vi "sha256.vi"(11 "data":string) -> (3 "sha256":u32[](array[numeric]) format="%08x")   [LabVIEW 2020, in "wamplv.lvlib" / "HashLib.lvclass"]
doc: "Calculates the <b>SHA-256</b> hash of the <b>data</b> input string.\n\nRFC 4634\n\nCreated by: Ryan Pacini"
uses:
  HashLib.lvclass
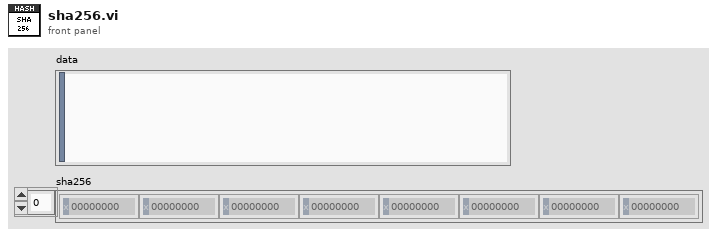
[diagram p1: front panel]
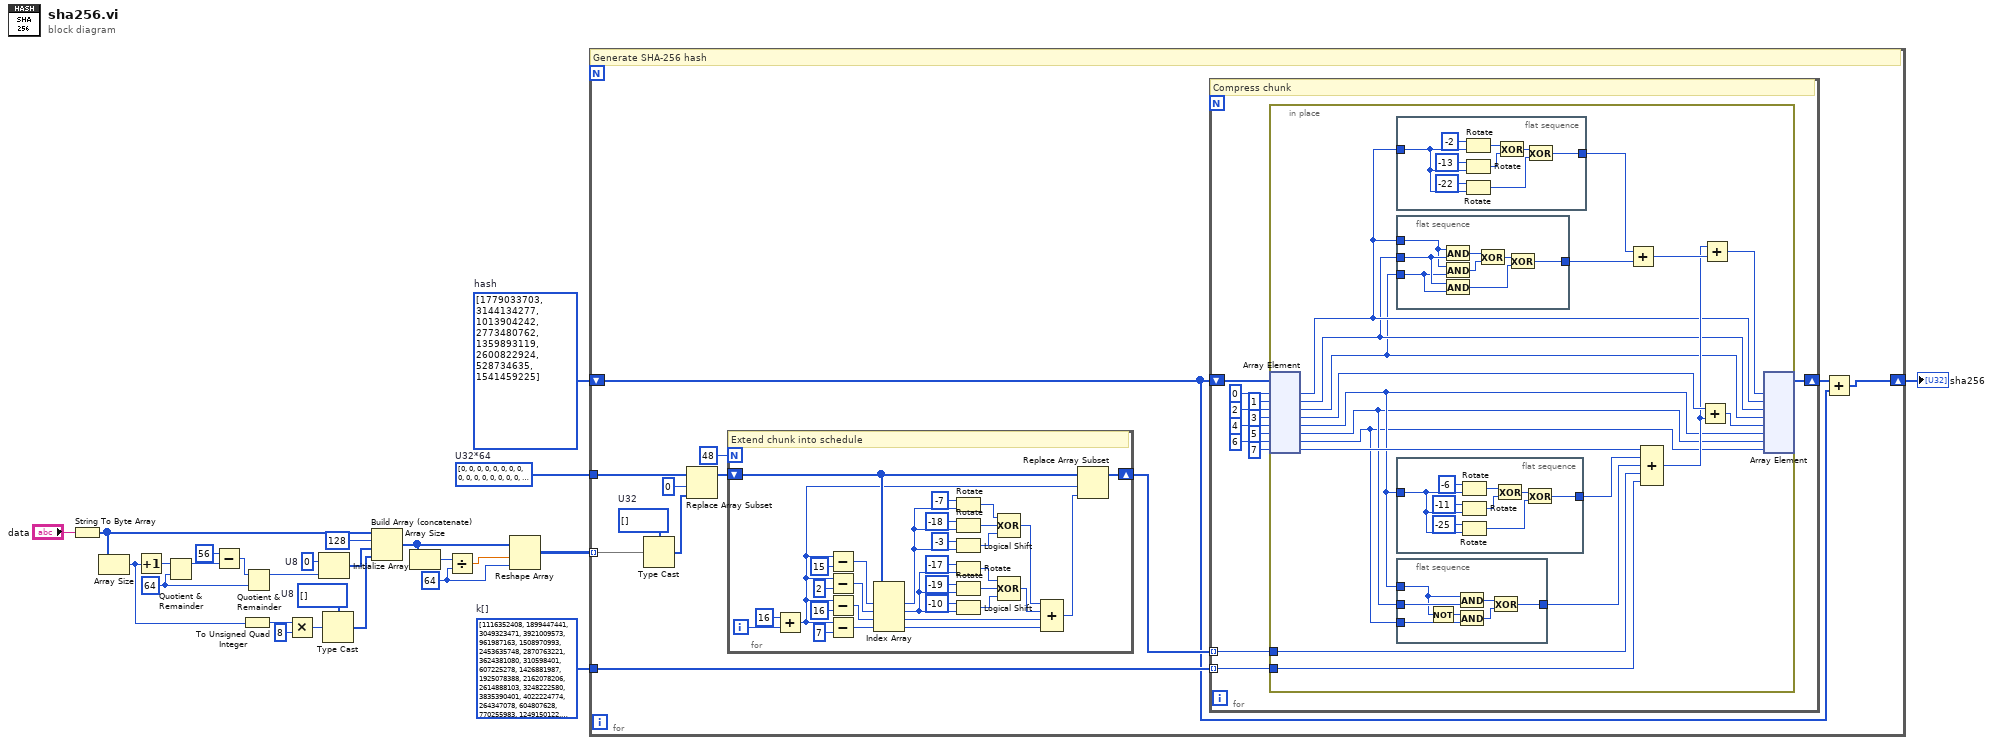
[diagram p0: block diagram]
diagram:
  w1 = u32[] [0, 0, 0, 0, 0, 0, 0, 0, 0, 0, 0, 0, 0, 0, 0, 0, 0, 0, 0, 0, 0, 0, 0, 0, 0, 0, 0, 0, 0, 0, 0, 0, 0, 0, 0, 0, 0, 0, 0, 0, 0, 0, 0, 0, 0, 0, 0, 0, 0, 0, 0, 0, 0, 0, 0, 0, 0, 0, 0, 0, 0, 0, 0, 0]  # U32*64
  w4 = 64
  w5 = u8[] []  # U8
  w18 = u8 0  # U8
  w3 = 64
  w23 = u32[] [1116352408, 1899447441, 3049323471, 3921009573, 961987163, 1508970993, 2453635748, 2870763221, 3624381080, 310598401, 607225278, 1426881987, 1925078388, 2162078206, 2614888103, 3248222580, 3835390401, 4022224774, 264347078, 604807628, 770255983, 1249150122, 1555081692, 1996064986, 2554220882, 2821834349, 2952996808, 3210313671, 3336571891, 3584528711, 113926993, 338241895, 666307205, 773529912, 1294757372, 1396182291, 1695183700, 1986661051, 2177026350, 2456956037, 2730485921, 2820302411, 3259730800, 3345764771, 3516065817, 3600352804, 4094571909, 275423344, 430227734, 506948616, 659060556, 883997877, 958139571, 1322822218, 1537002063, 1747873779, 1955562222, 2024104815, 2227730452, 2361852424, 2428436474, 2756734187, 3204031479, 3329325298]  # k[]
  w24 = u32[] [1779033703, 3144134277, 1013904242, 2773480762, 1359893119, 2600822924, 528734635, 1541459225]  # hash
  n1 = String To Byte Array(string="data") -> (unsigned byte array=w8:u8[])
  n2 = Array Size(array=w8) -> (size(s)=w11:i32)
  n3 = Increment(x=w11) -> (x+1=w21:i32)
  n4 = Quotient & Remainder(x=w21, y=w3) -> (x-y*floor(x/y)=w20:i32)  [unwired: 1 out]
  n5 = Subtract(x=56, y=w20) -> (x-y=w12:i32)
  n6 = To Unsigned Quad Integer(1:w11) -> (0:w10:u64)
  n7 = Quotient & Remainder(x=w12, y=w3) -> (x-y*floor(x/y)=w6:i32)  [unwired: 1 out]
  n8 = Multiply(x=w10, y=u64 8) -> (x*y=w2:u64)
  n9 = Initialize Array(w18, w6) -> (w17:u8[])
  n10 = Type Cast(type=w5, x=w2) -> (*(type *) &x=w7:u8[])
  n11 = Build Array (concatenate)(w8, u8 128, w17, w7) -> (w14:u8[])
  n12 = Array Size(array=w14) -> (size(s)=w15:i32)
  n13 = Divide(x=w15, y=w4) -> (x/y=w13:dbl)
  n14 = Reshape Array(w14, w13, w4) -> (w22:u8[][])
  n15 = for {
    tunnel: w22 -> [w38] mode=indexing
    tunnel: w1 -> [w36]
    tunnel: w23 -> [w31]
    shift-right: [w29] -> w25
    shift-left: w24 -> [w30]
    w37 = u32[] []  # U32
    # "Generate SHA-256 hash"
    n16 = Type Cast(type=w37, x=w38) -> (*(type *) &x=w35:u32[])
    n17 = Replace Array Subset(array=w36, new element=w35, index=0) -> (w33:u32[])
    n18 = for {
      N: 48 -> [_]
      shift-right: [w41] -> w32
      shift-left: w33 -> [w64]
      i -> [w70]
      # "Extend chunk into schedule"
      n19 = Add(x=16, y=w70) -> (x+y=w39:i32)
      n20 = Subtract(x=w39, y=15) -> (x-y=w68:i32)
      n21 = Subtract(x=w39, y=2) -> (x-y=w66:i32)
      n22 = Subtract(x=w39, y=16) -> (x-y=w63:i32)
      n23 = Subtract(x=w39, y=7) -> (x-y=w60:i32)
      n24 = Index Array(array=w64, index #1=w68, index #2=w66, index #3=w63, index #4=w60) -> (element #1=w57:u32, element #2=w50:u32, element #3=w43:u32, element #4=w42:u32)
      n25 = Rotate(1:w57, 2:i16 -7 ("y")) -> (0:w55:u32)
      n26 = Rotate(1:w57, 2:i16 -18 ("y")) -> (0:w54:u32)
      n27 = Logical Shift(y=i16 -3, x=w57) -> (x << y=w53:u32)
      n28 = Rotate(1:w50, 2:i16 -17 ("y")) -> (0:w46:u32)
      n29 = Rotate(1:w50, 2:i16 -19 ("y")) -> (0:w47:u32)
      n30 = Logical Shift(y=i16 -10, x=w50) -> (x << y=w48:u32)
      n31 = Compound Arithmetic op=XOR(w55, w54, w53) -> (w45:u32)
      n32 = Compound Arithmetic op=XOR(w46, w47, w48) -> (w44:u32)
      n33 = Compound Arithmetic op=ADD(w45, w44, w43, w42) -> (w40:u32)
      n34 = Replace Array Subset(array=w64, new element=w40, index=w39) -> (w41:u32[])
    }
    n35 = for {
      tunnel: w32 -> [w73] mode=indexing
      tunnel: w31 -> [w72] mode=indexing
      shift-right: [w71] -> w27
      shift-left: w30 -> [w82]
      # "Compress chunk"
      n36 = in-place {
        in-place-border: w73 -> [w99]
        in-place-border: w72 -> [w98]
        n37 = in-place-array #1(w82, 0, 1, 2, 3, 4, 5, 6, 7) -> (w91:u32, w90:u32, w89:u32, w97:u32, w86:u32, w85:u32, w84:u32, w100:u32)
        n38 = flat-sequence {
          tunnel: w91 -> [w130]
          tunnel: [w125] -> w92
          frame #0 {
            n39 = Rotate(1:w130, 2:i16 -2 ("y")) -> (0:w129:u32)
            n40 = Rotate(1:w130, 2:i16 -13 ("y")) -> (0:w128:u32)
            n41 = Rotate(1:w130, 2:i16 -22 ("y")) -> (0:w126:u32)
            n42 = Exclusive Or(1:w128, 2:w129) -> (0:w127:u32)
            n43 = Exclusive Or(1:w126, 2:w127) -> (0:w125:u32)
          }
        }
        n44 = flat-sequence {
          tunnel: w90 -> [w124]
          tunnel: w89 -> [w123]
          tunnel: w91 -> [w122]
          tunnel: [w117] -> w88
          frame #0 {
            n45 = And(x=w122, y=w124) -> (x .and. y?=w121:u32)
            n46 = And(x=w122, y=w123) -> (x .and. y?=w120:u32)
            n47 = And(x=w124, y=w123) -> (x .and. y?=w118:u32)
            n48 = Exclusive Or(1:w120, 2:w121) -> (0:w119:u32)
            n49 = Exclusive Or(1:w118, 2:w119) -> (0:w117:u32)
          }
        }
        n50 = flat-sequence {
          tunnel: w86 -> [w113]
          tunnel: [w108] -> w87
          frame #0 {
            n51 = Rotate(1:w113, 2:i16 -6 ("y")) -> (0:w112:u32)
            n52 = Rotate(1:w113, 2:i16 -11 ("y")) -> (0:w111:u32)
            n53 = Rotate(1:w113, 2:i16 -25 ("y")) -> (0:w109:u32)
            n54 = Exclusive Or(1:w111, 2:w112) -> (0:w110:u32)
            n55 = Exclusive Or(1:w109, 2:w110) -> (0:w108:u32)
          }
        }
        n56 = flat-sequence {
          tunnel: w85 -> [w107]
          tunnel: w86 -> [w106]
          tunnel: w84 -> [w104]
          tunnel: [w101] -> w83
          frame #0 {
            n57 = Not(x=w106) -> (.not. x?=w105:u32)
            n58 = And(x=w106, y=w107) -> (x .and. y?=w103:u32)
            n59 = And(x=w105, y=w104) -> (x .and. y?=w102:u32)
            n60 = Exclusive Or(1:w102, 2:w103) -> (0:w101:u32)
          }
        }
        n61 = Add(x=w92, y=w88) -> (x+y=w95:u32)
        n62 = Compound Arithmetic op=ADD(w100, w87, w83, w99, w98) -> (w93:u32)
        n63 = Add(x=w97, y=w93) -> (x+y=w96:u32)
        n64 = Add(x=w93, y=w95) -> (x+y=w94:u32)
        n65 = in-place-array #1(w94, w91, w90, w89, w96, w86, w85, w84) -> (w71:u32[])  [unwired: 8 out]
      }
    }
    n66 = Add(x=w27, y=w30) -> (x+y=w29:u32[])
  }
  "sha256" <- w25
